vi "caxis_rough_fit.vi"(8 "Error In":errorcluster, 11 "Sample Results":T1) -> (0 "Error Out":errorcluster, 1 "Best R2":dbl[](array[numeric]), 2 "Theta min":dbl[](array[numeric]), 3 "Phi min":dbl[](array[numeric]))   [LabVIEW 2019]
uses:
  sample_results_cluster_typedef.ctl
  parameters_cluster_typedef.ctl
  writeable_section_parameters_cluster_typedef.ctl
  grain_results_cluster_typedef.ctl
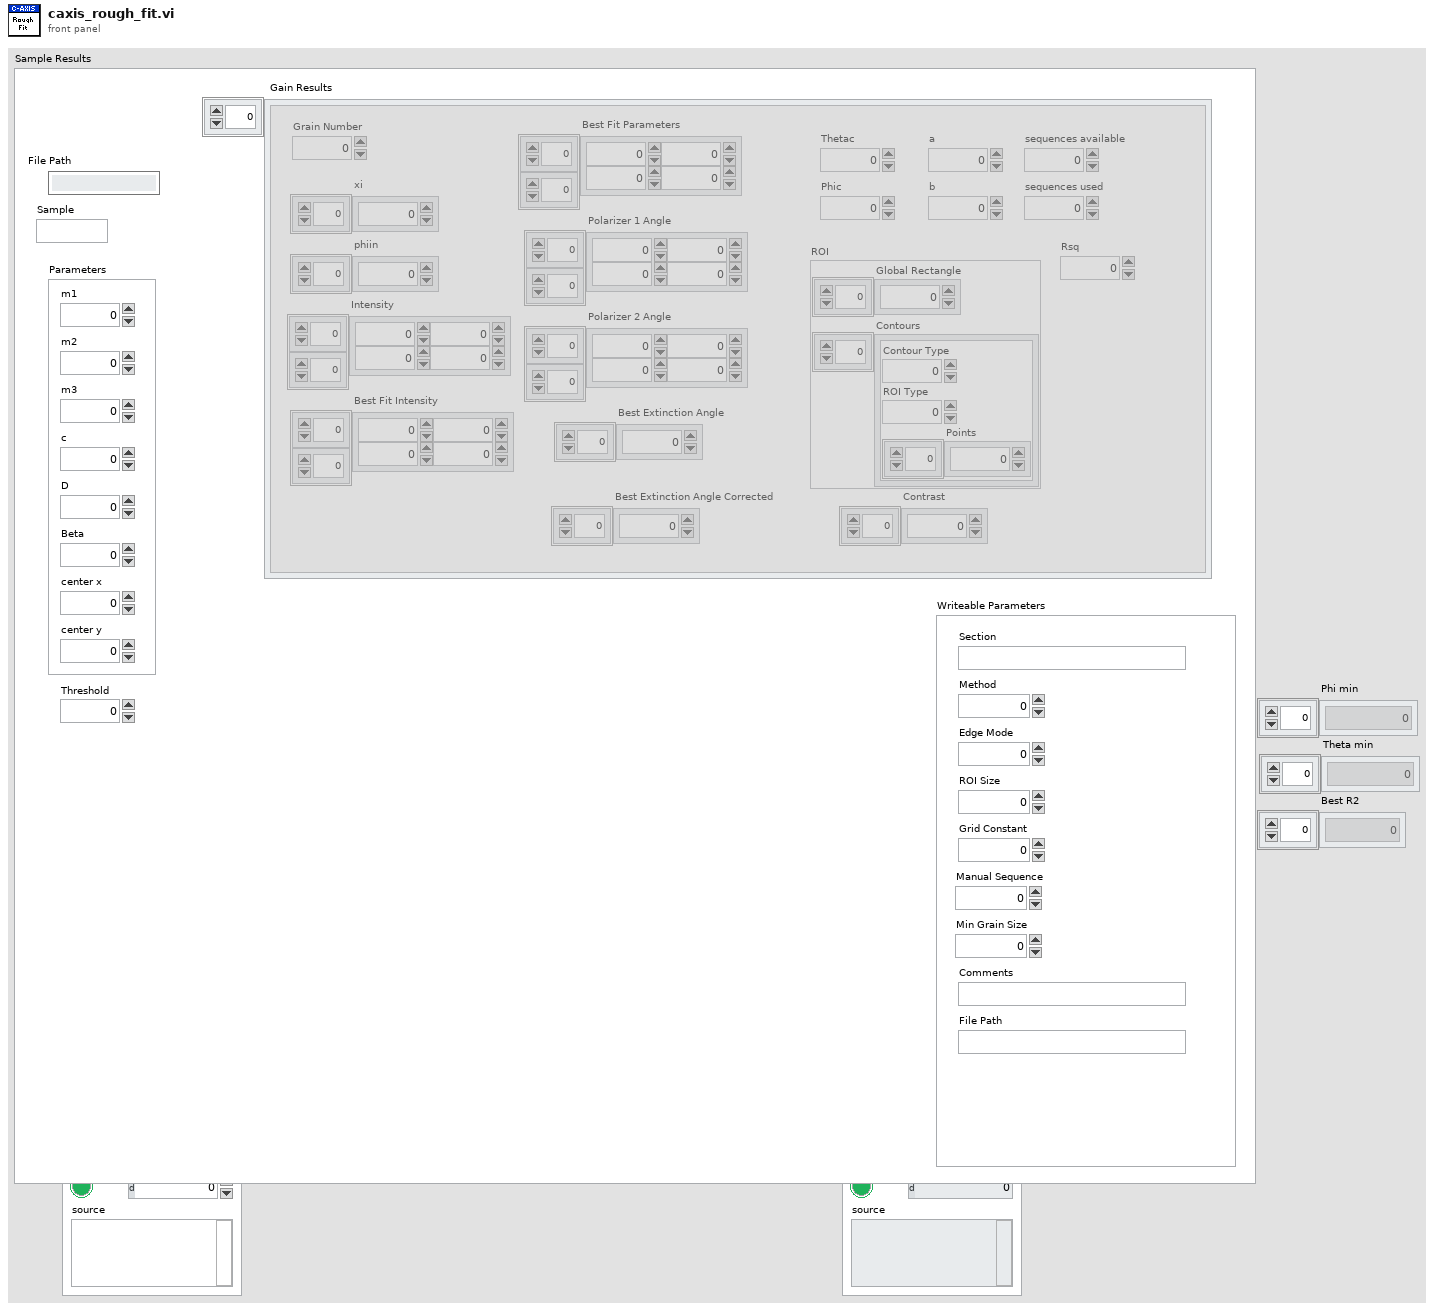
[diagram p1: front panel]
types:
  T1 = typedef "sample_results_cluster_typedef.ctl" = cluster{"File Path":string, "Sample":string, "Threshold":dbl, "Parameters":T2, "Writeable Parameters":T3, "Gain Results":T4[]}
  T2 = typedef "parameters_cluster_typedef.ctl" = cluster{"m1":dbl, "m2":dbl, "m3":dbl, "c":dbl, "D":dbl, "Beta":dbl, "center x":dbl, "center y":dbl}
  T3 = typedef "writeable_section_parameters_cluster_typedef.ctl" = cluster{"Section":string, "Method":i32, "Edge Mode":i32, "Grid Constant":i32, "Manual Sequence":i32, "ROI Size":i32, "Min Grain Size":dbl, "Comments":string, "File Path":string}
  T4 = typedef "grain_results_cluster_typedef.ctl" = cluster{"Grain Number":i32, "xi":dbl[], "phiin":dbl[], "Intensity":dbl[][], "Best Fit Intensity":dbl[][], "Best Fit Parameters":dbl[][], "Polarizer 1 Angle":dbl[][], "Polarizer 2 Angle":dbl[][], "Best Extinction Angle":dbl[], "Best Extinction Angle Corrected":dbl[], "Thetac":dbl, "Phic":dbl, "ROI":cluster{"Global Rectangle":i32[], "Contours":cluster{"Contour Type":u32, "ROI Type":u32, "Points":i32[]}[]}, "a":dbl, "b":dbl, "sequences available":dbl, "sequences used":dbl, "Contrast":dbl[], "Rsq":dbl}
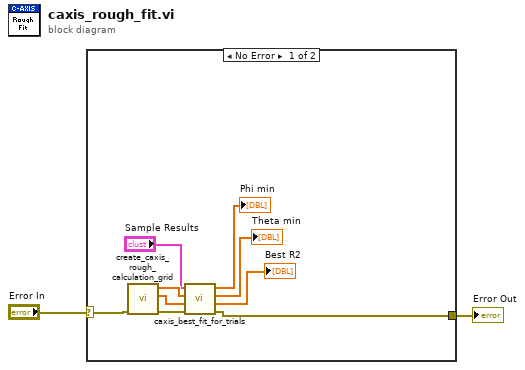
[diagram p0: block diagram]
diagram:
  n1 = case shown="No Error" "Error In" {
    selector: "Error In" -> [w11 w12]
    tunnel: [w6 w12] -> w1
    frame No Error {
      n2 = call "create_caxis_rough_calculation_grid.vi"("Error In"=w11) -> ("Error Out"=w8:errorcluster, "phic"=w9:dbl[], "thetac"=w10:dbl[])  [unwired: 8 in]
      n3 = call "caxis_best_fit_for_trials.vi"("Error In"=w8, "phic"=w9, "thetac"=w10, "Sample Results"="Sample Results") -> ("Error Out"=w6:errorcluster, "Best R2"=→"Best R2":dbl[], "Theta min"=→"Theta min":dbl[], "Phi min"=→"Phi min":dbl[])  [unwired: 4 in]
    }
    frame Error {
    }
  }
  "Error Out" <- w1
